vi "Query CV CC.vi"(7 "Slave Address":i32=-1 min=-1 max=30 step=1, 8 "error":errorcluster, 11 "VISA":refnum<visa-resource-name>) -> (0 "error out":errorcluster, 1 "CC":bool, 2 "CV":bool, 3 "VISA out":refnum<visa-resource-name>, 4 "Mode":enum16{"OFF", "CV", "CC"}(ring), 5 "Output ON":bool)   [LabVIEW 2025, in "TDK-Lambda GEN LAN Series.lvlib"]
doc: "Returns the operating mode of the power supply:\n\n\"CV\" is TRUE if in Constant Voltage mode\n\"CC\" is TRUE if in Constant Current mode\n\"Output ON\" is TRUE if the output is ON\n\"Mode\" is an enumerated type with values \"OFF\", \"CV\" or \"CC\"."
uses:
  <userlib>/TDK-Lambda GEN LAN Series/TDK-Lambda GEN LAN Series.lvlib
panel:
  # "TDK-Lambda Genesys \n LAN\n  DC Power Supplies"
  # "Read Condition:\n  CV, CC or OFF"
  # "(c) 2019 TDK-Lambda.  ALL RIGHTS RESERVED."
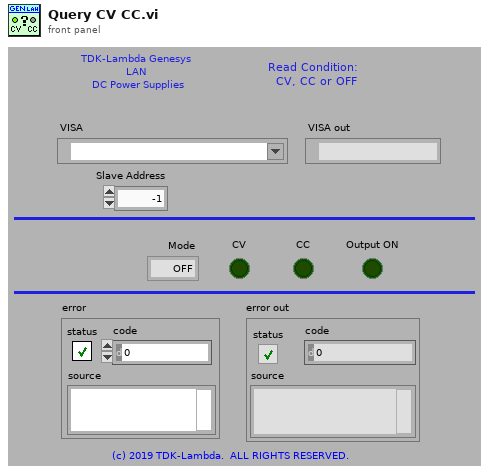
[diagram p1: front panel]
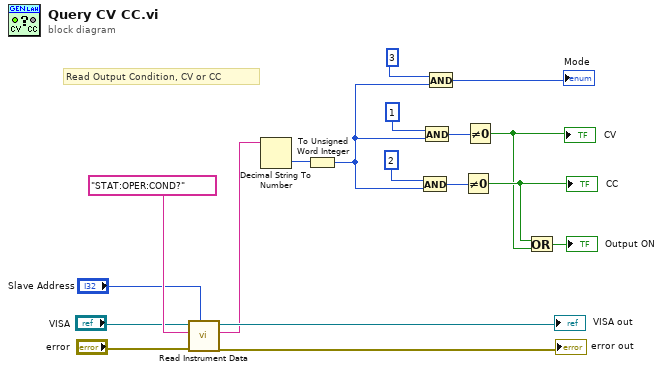
[diagram p0: block diagram]
diagram:
  # "Read Output Condition, CV or CC"
  n1 = call <userlib>:"Read Instrument Data.vi"("Slave Address"="Slave Address", "error"="error", "Query"="STAT:OPER:COND?" ("format string"), "VISA"="VISA") -> ("error out"=→"error out":errorcluster, "Response"=w15:string, "VISA out"=→"VISA out":refnum<visa-resource-name>)  [unwired: 4 in, 1 out]
  n2 = Decimal String To Number(string=w15) -> (number=w14:i32)  [unwired: 2 in, 1 out]
  n3 = To Unsigned Word Integer(number=w14) -> (unsigned 16bit integer=w3:u16)
  n4 = And(x=u16 2, y=w3) -> (x .and. y?=w11:u16)
  n5 = And(x=u16 1, y=w3) -> (x .and. y?=w12:u16)
  n6 = And(x=u16 3 ("Numeric"), y=w3) -> (x .and. y?=→"Mode":u16)
  n7 = Not Equal To 0?(x=w11) -> (x != 0?=w8:bool)
  "CC" <- w8
  n8 = Not Equal To 0?(x=w12) -> (x != 0?=w7:bool)
  "CV" <- w7
  n9 = Or(x=w8, y=w7) -> (x .or. y?=→"Output ON":bool)
